vi "Get image delay.vi"(8 "error in (no error)":errorcluster, 11 "CCDCamera in":refnum<class "CCDCamera.lvclass">) -> (0 "error out":errorcluster, 3 "CCDCamera out":refnum<class "CCDCamera.lvclass">)   [LabVIEW 2018, in "CCDCamera.lvclass"]
doc: "Get the delay of the start of an exposure from the start of a kinetic series.\n\nThis function should only be used in a kinetic series with two or more frames."
uses:
  CCDCamera.lvclass
  C:/Users/observer/Desktop/SPARC4_ACS/SPARC4_ACS/Simulated_CCD_Camera/Simulated_CCD_Camera.lvclass
  Simulated_CCD_Camera/Simulated_CCD_Camera.lvclass
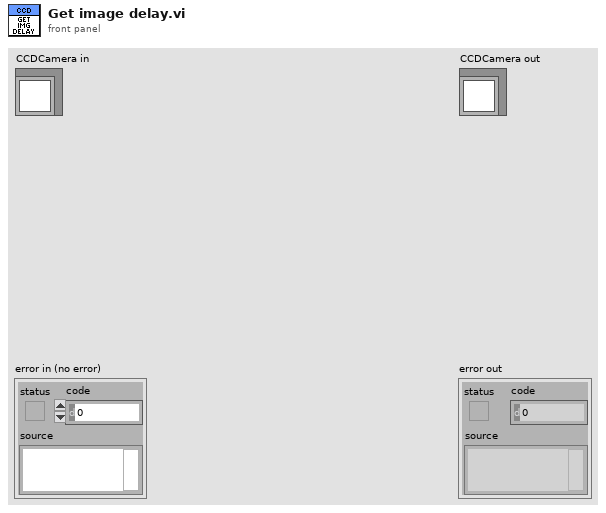
[diagram p1: front panel]
types:
  T1 = cluster{"CYCLES_DONE":u16, "LAST_IMAGE_NAME":string, "DISK_SPACE":u16, "FRAMES_DONE":u16, "CCD_STATUS":string, "CURRENT_TEMPERATURE":i16, "TEMPERATURE_STATUS":string, "FRAME_EXPOSURE_TIME":sgl, "ERROR":bool, "SERIAL_NUMBER":u16, "ACQUIRING":bool, "IMAGE_INDEX":u32, "SEQS_DONE":u16}
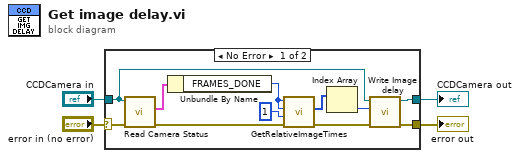
[diagram p0: block diagram]
diagram:
  n1 = case shown="No Error" "error in (no error)" {
    selector: "error in (no error)" -> [w9 w16]
    tunnel: "CCDCamera in" -> [w7 w17]
    tunnel: [w15 w17] -> w2
    tunnel: [w14 w16] -> w1
    frame No Error {
      n2 = call "Read Camera Status.vi"("error in (no error)"=w9, "CCDCamera in"=w7) -> ("error out"=w8:errorcluster, "Camera Status"=w6:T1)  [unwired: 7 in, 1 out]
      n3 = Unbundle By Name(w6) -> ("FRAMES_DONE"=w5:u16)
      n4 = call <userlib>:"GetRelativeImageTimes.vi"("error in (no error)"=w8, "size"=u32 1 ("first"), "last"=w5, "first"=w5) -> ("error out"=w11:errorcluster, "arr"=w12:u64[])  [unwired: 5 in, 1 out]
      n5 = Index Array(array=w12) -> (element=w10:u64)  [unwired: 1 in]
      n6 = call-dynamic "Write Image delay.vi"("error in (no error)"=w11, "Image delay"=w10, "Simulated_CCD_Camera in"=w7) -> ("error out"=w14:errorcluster, "Simulated_CCD_Camera out"=w15:refnum<class "CCDCamera.lvclass">)  [unwired: 7 in]
    }
    frame Error {
    }
  }
  "error out" <- w1
  "CCDCamera out" <- w2
